vi "Initialize Dispenser.vi"(8 "error in":errorcluster, 11 "Gantry in":refnum<class "Gantry Class.lvclass">) -> (0 "error out":errorcluster, 3 "Gantry out":refnum<class "Gantry Class.lvclass">)   [LabVIEW 2017, in "Gantry Class.lvclass"]
uses:
  Gantry Class.lvclass
  Gantry Class.lvclass/Gantry Class.ctl
  <vilib>/DAQmx/write.llb/DAQmx Write (Digital Bool 1Line 1Point).vi
  <vilib>/DAQmx/create/channels.llb/DAQmx Create Channel (DO-Digital Output).vi
  <vilib>/DAQmx/miscellaneous.llb/DAQmx Fill In Error Info.vi
  FlexWorktable/FlexWorktable.lvclass
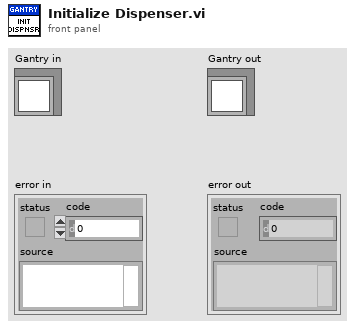
[diagram p1: front panel]
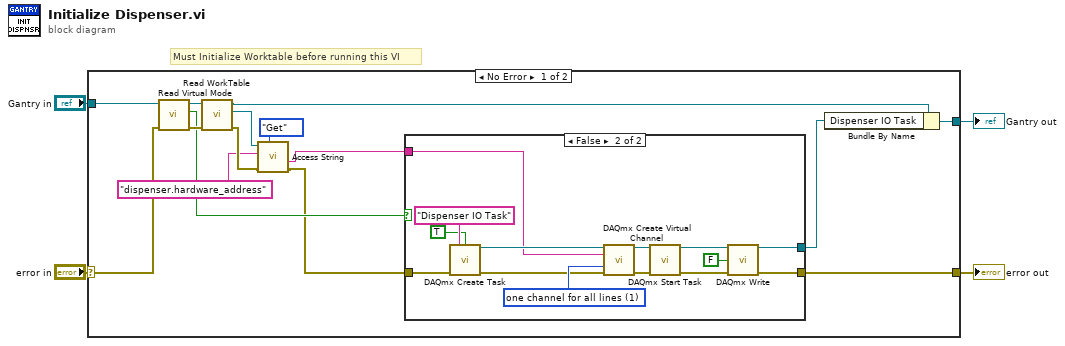
[diagram p0: block diagram]
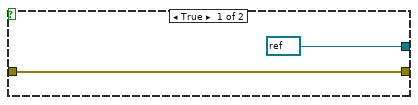
[diagram p2: hidden frame]
diagram:
  # "Must Initialize Worktable before running this VI"
  n1 = case shown="No Error" "error in" {
    selector: "error in" -> [w12 w37]
    tunnel: [w17 w37] -> w2
    tunnel: [w18 w36] -> w1
    tunnel: "Gantry in" -> [w15 w36]
    frame No Error {
      n2 = call-dynamic "Read Virtual Mode.vi"("error in (no error)"=w12, "Gantry in"=w15) -> ("error out"=w13:errorcluster, "Is Virtual"=w11:bool, "Gantry out"=w14:refnum<class "Gantry Class.lvclass">)  [unwired: 6 in, 1 out]
      n3 = call-dynamic "Read WorkTable.vi"("error in"=w13, "Gantry Class in"=w14) -> ("error out"=w9:errorcluster, "Worktable"=w10:refnum<class "FlexWorktable.lvclass">, "Gantry Class out"=w19:refnum<class "Gantry Class.lvclass">)  [unwired: 7 in]
      n4 = call-dynamic "Access String.vi"("Get/Set"=enum16{"Get", "Set"}."Get", "error in (no error)"=w9, "Key"="dispenser.hardware_address", "FlexWorktable in"=w10) -> ("error out"=w8:errorcluster, "Value out"=w5:string)  [unwired: 5 in, 1 out]
      n5 = case shown="False" w11 {
        tunnel: [w21 w24] -> w17
        tunnel: [refnum<k21> refnum ("task out") w23] -> w16
        tunnel: w5 -> [_ w29]
        tunnel: w8 -> [w21 w27]
        frame True {
        }
        frame False {
          w30 = 1 items=["one channel for each line", "one channel for all lines"] ("line grouping")
          n6 = call <vilib>:"DAQmx Create Task.vi"("new task name"="Dispenser IO Task", "auto cleanup"=TRUE, "error in"=w27) -> ("task out"=w31:refnum<k21>, "error out"=w28:errorcluster)  [unwired: 2 in, 9 out]
          n7 = call-poly <vilib>:"DAQmx Create Virtual Channel.vi"("task in"=w31, "lines"=w29, "line grouping"=w30, "error in"=w28) -> ("task out"=w33:refnum<k21>, "error out"=w32:errorcluster)  [unwired: 1 in, 9 out]
          n8 = call <vilib>:"DAQmx Start Task.vi"("task/channels in"=w33, "error in"=w32) -> ("task out"=w26:refnum<k21>, "error out"=w25:errorcluster)  [unwired: 12 out]
          n9 = call-poly <vilib>:"DAQmx Write.vi"("task/channels in"=w26, "data"=FALSE, "error in"=w25) -> ("task out"=w23:refnum<k21>, "error out"=w24:errorcluster)  [unwired: 10 in, 1 out]
        }
      }
      n10 = Bundle By Name(cluster=w19, "Dispenser IO Task"=w16) -> (w18:refnum<class "Gantry Class.lvclass">)
    }
    frame Error {
    }
  }
  "error out" <- w2
  "Gantry out" <- w1
